vi "Config Conflict Zones.vi"(8 "error in (no error)":errorcluster, 11 "Configuration in":refnum<class "Configuration.lvclass">) -> (0 "error out":errorcluster, 3 "Configuration out":refnum<class "Configuration.lvclass">)   [LabVIEW 2016, in "Hardware.lvlib" / "VacuumLine.lvlib" / "VacuumLines Configuration.lvclass"]
uses:
  <userlib>/Common Components/Hardware/Abstract System/VacuumLine/VacuumLines Configuration/VacuumLines Configuration.lvclass
  <userlib>/Configuration Dialog Actor/Configuration.lvclass
  <userlib>/Common Components/Hardware/Abstract System/VacuumLine/VacuumLines/Conflict Zone.ctl
  C:/Program Files (x86)/National Instruments/LabVIEW 2016/user.lib/Configuration Dialog Actor/Configuration.lvclass
  <userlib>/Common Components/Hardware/Abstract System/VacuumLine/VacuumLines Configuration/VacuumLines Configuration.lvclass/VacuumLines Configuration.ctl
  <userlib>/Common Components/Hardware/Abstract System/VacuumLine/VacuumLines/VacuumLines.lvclass
panel:
  in  "No. of Conflict Zones":u8
  in  "Array of Conflict Zones":T1[](array[typedef]) caption="Conflict Zones (unit in mm)"
  in  "Revert":bool
  in  "Apply":bool
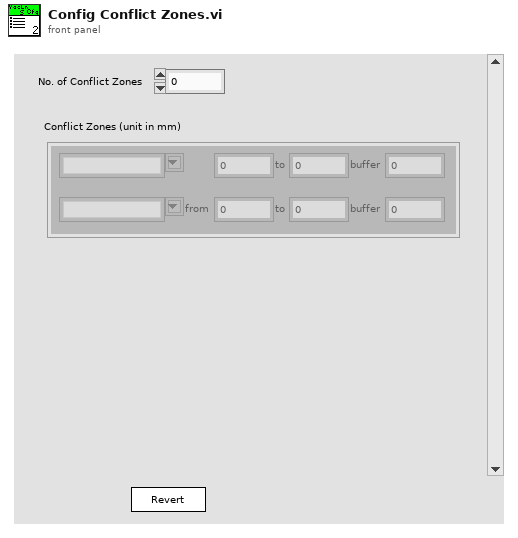
[diagram p1: front panel]
types:
  T1 = typedef "Hardware.lvlib/VacuumLine.lvlib/VacuumLines.lvclass/Conflict Zone.ctl" = cluster{"1":cluster{"Label":string, "from":dbl, "to":dbl, "buffer":dbl}, "2":cluster{"Label":string, "from":dbl, "to":dbl, "buffer":dbl}}
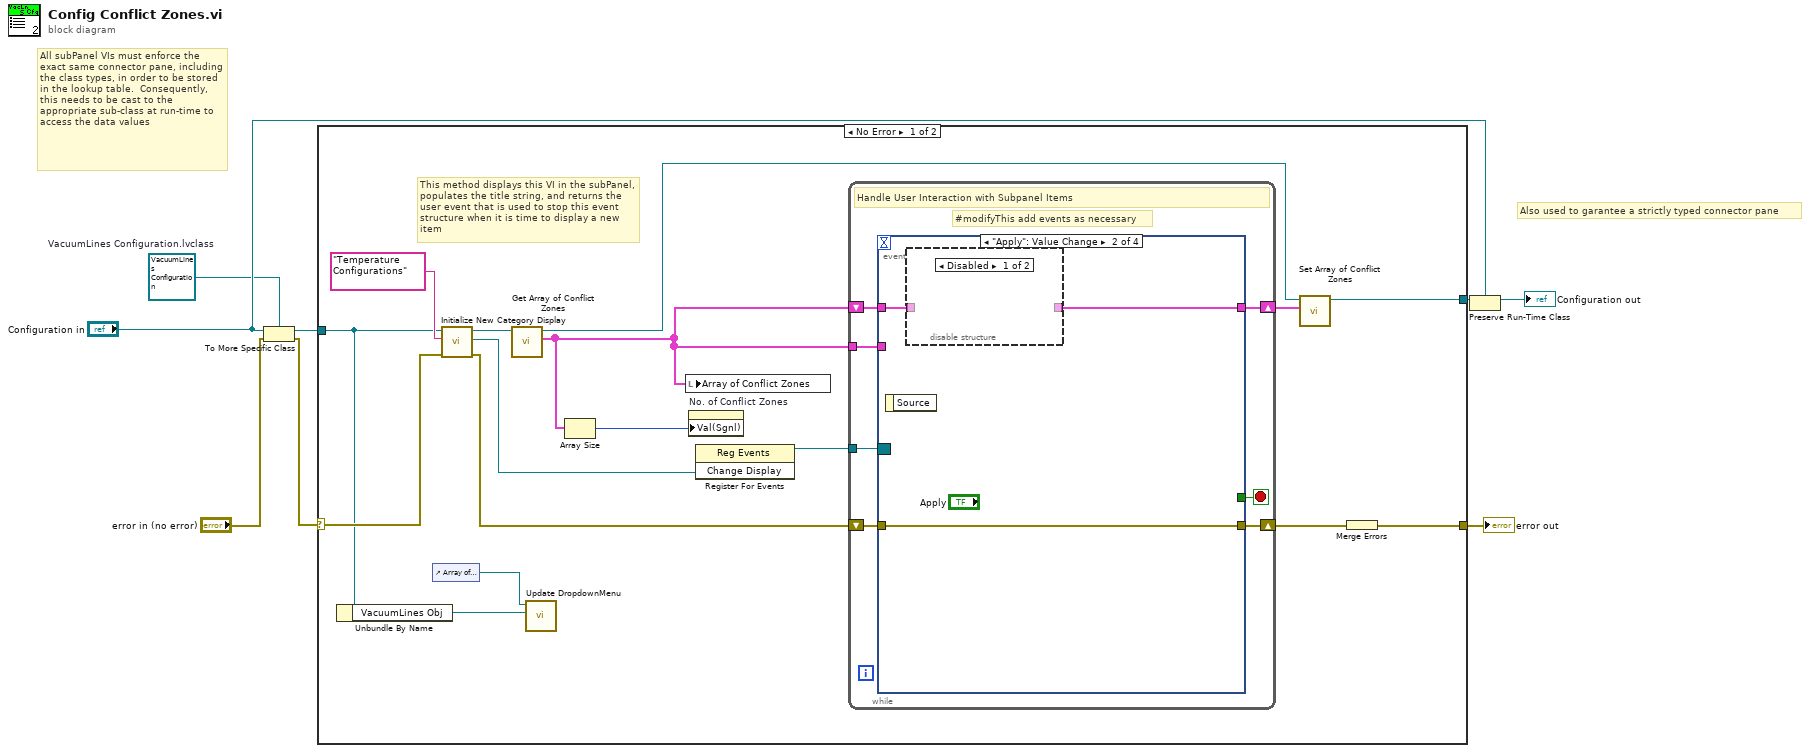
[diagram p0: block diagram]
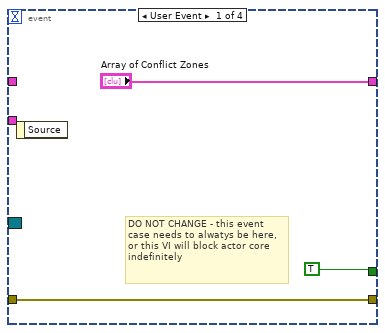
[diagram p2: hidden frame]
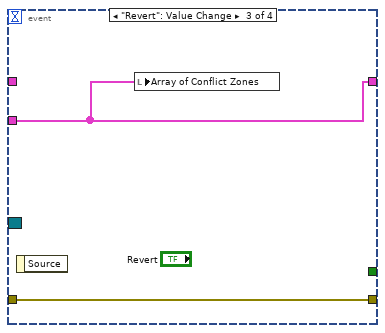
[diagram p4: hidden frame]
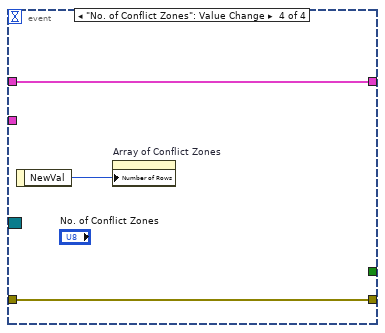
[diagram p5: hidden frame]
diagram:
  w2 = refnum<class "VacuumLines Configuration.lvclass"> refnum  # VacuumLines Configuration.lvclass
  # "Also used to garantee a strictly typed connector pane"
  # "All subPanel VIs must enforce the exact same connector pane, including the class types, in order to be stored in the lookup table.  Consequently, this needs to be cast to the appropriate sub-class at run-time to access the data values"
  n1 = To More Specific Class(target class=w2, reference="Configuration in", error in="error in (no error)") -> (specific class reference=w6:refnum<class "VacuumLines Configuration.lvclass">, error out=w1:errorcluster)
  n2 = case shown="No Error" w1 {
    selector: w1 -> [w18 w44]
    tunnel: w6 -> [w12 w45]
    tunnel: [w15 w45] -> w8
    tunnel: [w24 w44] -> w7
    frame No Error {
      # "This method displays this VI in the subPanel, populates the title string, and returns the user event that is used to stop this event structure when it is time to display a new item"
      n3 = Unbundle By Name(w12) -> ("VacuumLines Obj"=w11:refnum<class "VacuumLines.lvclass">)
      n4 = control-ref of="Array of Conflict Zones"() -> (w10:refnum<vi>)
      n5 = call <userlib>:"Initialize New Category Display.vi"("error in (no error)"=w18, "Name to Display"="Temperature Configurations", "Configuration in"=w12) -> ("error out"=w19:errorcluster, "Change Display"=w22:refnum<user-event>, "Configuration Out"=w17:refnum<class "VacuumLines Configuration.lvclass">)  [unwired: 6 in]
      n6 = call <userlib>:"Get Array of Conflict Zones.vi"("VacuumLines Configuration in"=w17) -> ("Array of Conflict Zones"=w13:T1[], "VacuumLines Configuration out"=w16:refnum<class "VacuumLines Configuration.lvclass">)  [unwired: 8 in, 1 out]
      n7 = call <userlib>:"Update DropdownMenu.vi"("VacuumLines Obj"=w11, "Ref of Array"=w10) -> ()  [unwired: 10 in]
      n8 = Array Size(array=w13) -> (size(s)=w9:i32)
      n9 = local write "Array of Conflict Zones"(w13) -> ()
      n10 = property on="No. of Conflict Zones" class="DigNum (strict)"("Val(Sgnl)"=w9) -> ()  [unwired: 2 in, 2 out]
      n11 = register-events(w22) -> (reference out=w21:refnum<event-registration>)  [unwired: 2 in, 1 out]
      n12 = while {
        tunnel: w21 -> [w30]
        shift-right: [w29] -> w20
        shift-left: w19 -> [w28]
        shift-right: [w26] -> w14
        shift-left: w13 -> [w27]
        tunnel: w13 -> [w25]
        stop <- w31 stop-if-true
        # "#modifyThis add events as necessary"
        # "Handle User Interaction with Subpanel Items"
        n13 = event shown="[1] \"Apply\": Value Change" {
          selector: w30 -> [_ _ _ _]
          dyn-events: _ -> [_ _ _ _]
          timeout: _ -> [_ _ _ _]
          tunnel: [TRUE _ _ _] -> w31
          tunnel: [w34 w37 w40 w43] -> w29
          tunnel: w28 -> [w34 w37 w40 w43]
          tunnel: w27 -> [_ w35 _ w42]
          tunnel: ["Array of Conflict Zones" w36 w39 w42] -> w26
          tunnel: w25 -> [_ _ w39 _]
          event User Event {
            # "DO NOT CHANGE - this event case needs to alwatys be here, or this VI will block actor core indefinitely"
            n14 = event-data() -> ()  [unwired: 1 in, 1 out]
          }
          event "Apply": Value Change {
            n15 = event-data() -> ()  [unwired: 1 in, 1 out]
            n16 = disable-structure shown="Disabled" {
              disable-tunnel: [_ w38] -> w36
              disable-tunnel: w35 -> [_ w38]
              frame Disabled {
              }
              frame Enabled {
              }
            }
          }
          event "Revert": Value Change {
            n17 = event-data() -> ()  [unwired: 1 in, 1 out]
            n18 = local write "Array of Conflict Zones"(w39) -> ()
          }
          event "No. of Conflict Zones": Value Change {
            n19 = event-data() -> ("NewVal"=w41:u8)  [unwired: 1 in]
            n20 = property on="Array of Conflict Zones" class="Arr (strict)"("Number of Rows"=w41) -> ()  [unwired: 2 in, 2 out]
          }
        }
      }
      n21 = call <userlib>:"Set Array of Conflict Zones.vi"("Array of Conflict Zones"=w14, "VacuumLines Configuration in"=w16) -> ("VacuumLines Configuration out"=w15:refnum<class "VacuumLines Configuration.lvclass">)  [unwired: 8 in, 1 out]
      n22 = Merge Errors(w20) -> (w24:errorcluster)
    }
    frame Error {
    }
  }
  "error out" <- w7
  n23 = Preserve Run-Time Class(object in=w8, 2:"Configuration in") -> (object out=→"Configuration out":refnum<class "Configuration.lvclass">)  [unwired: 1 in, 1 out]
